vi "wrl_import_Ex.vi"() -> ()   [LabVIEW 2020]
uses:
  <vilib>/picture/3D Picture Control/Object/Create Object (name).vi
  Interface.vi
  <vilib>/picture/3D Picture Control/NI_3D Picture Control.lvlib
panel:
  out "3D 그림":refnum<vi>(3d-picture)
  in  "bkt angle":dbl
  in  "arm angle":dbl=0.07999999821186066
  in  "boom angle":dbl
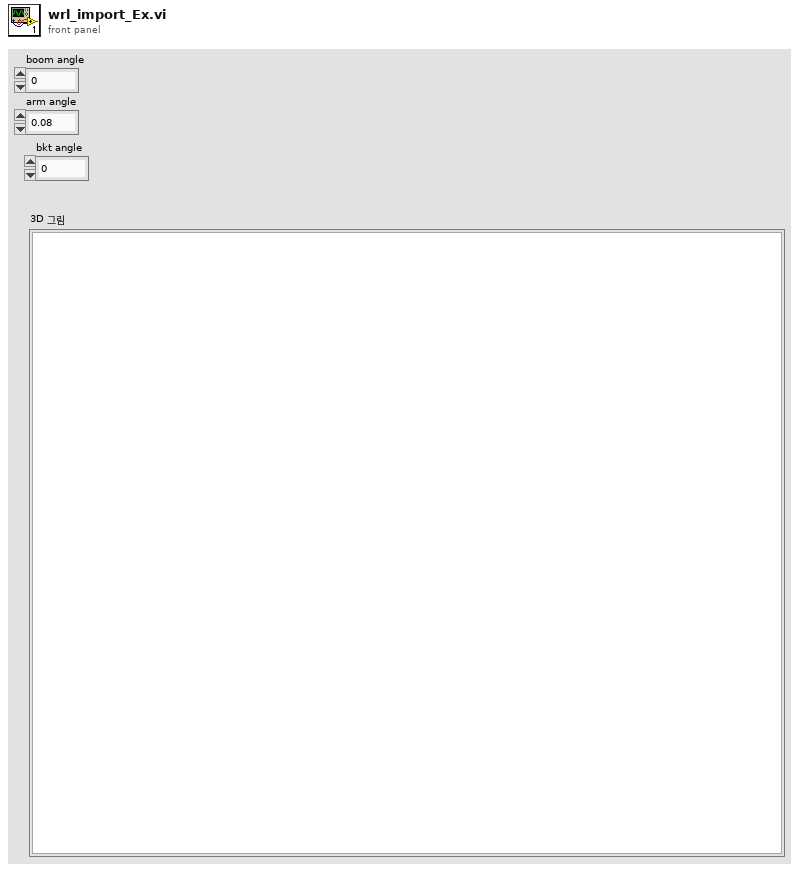
[diagram p1: front panel]
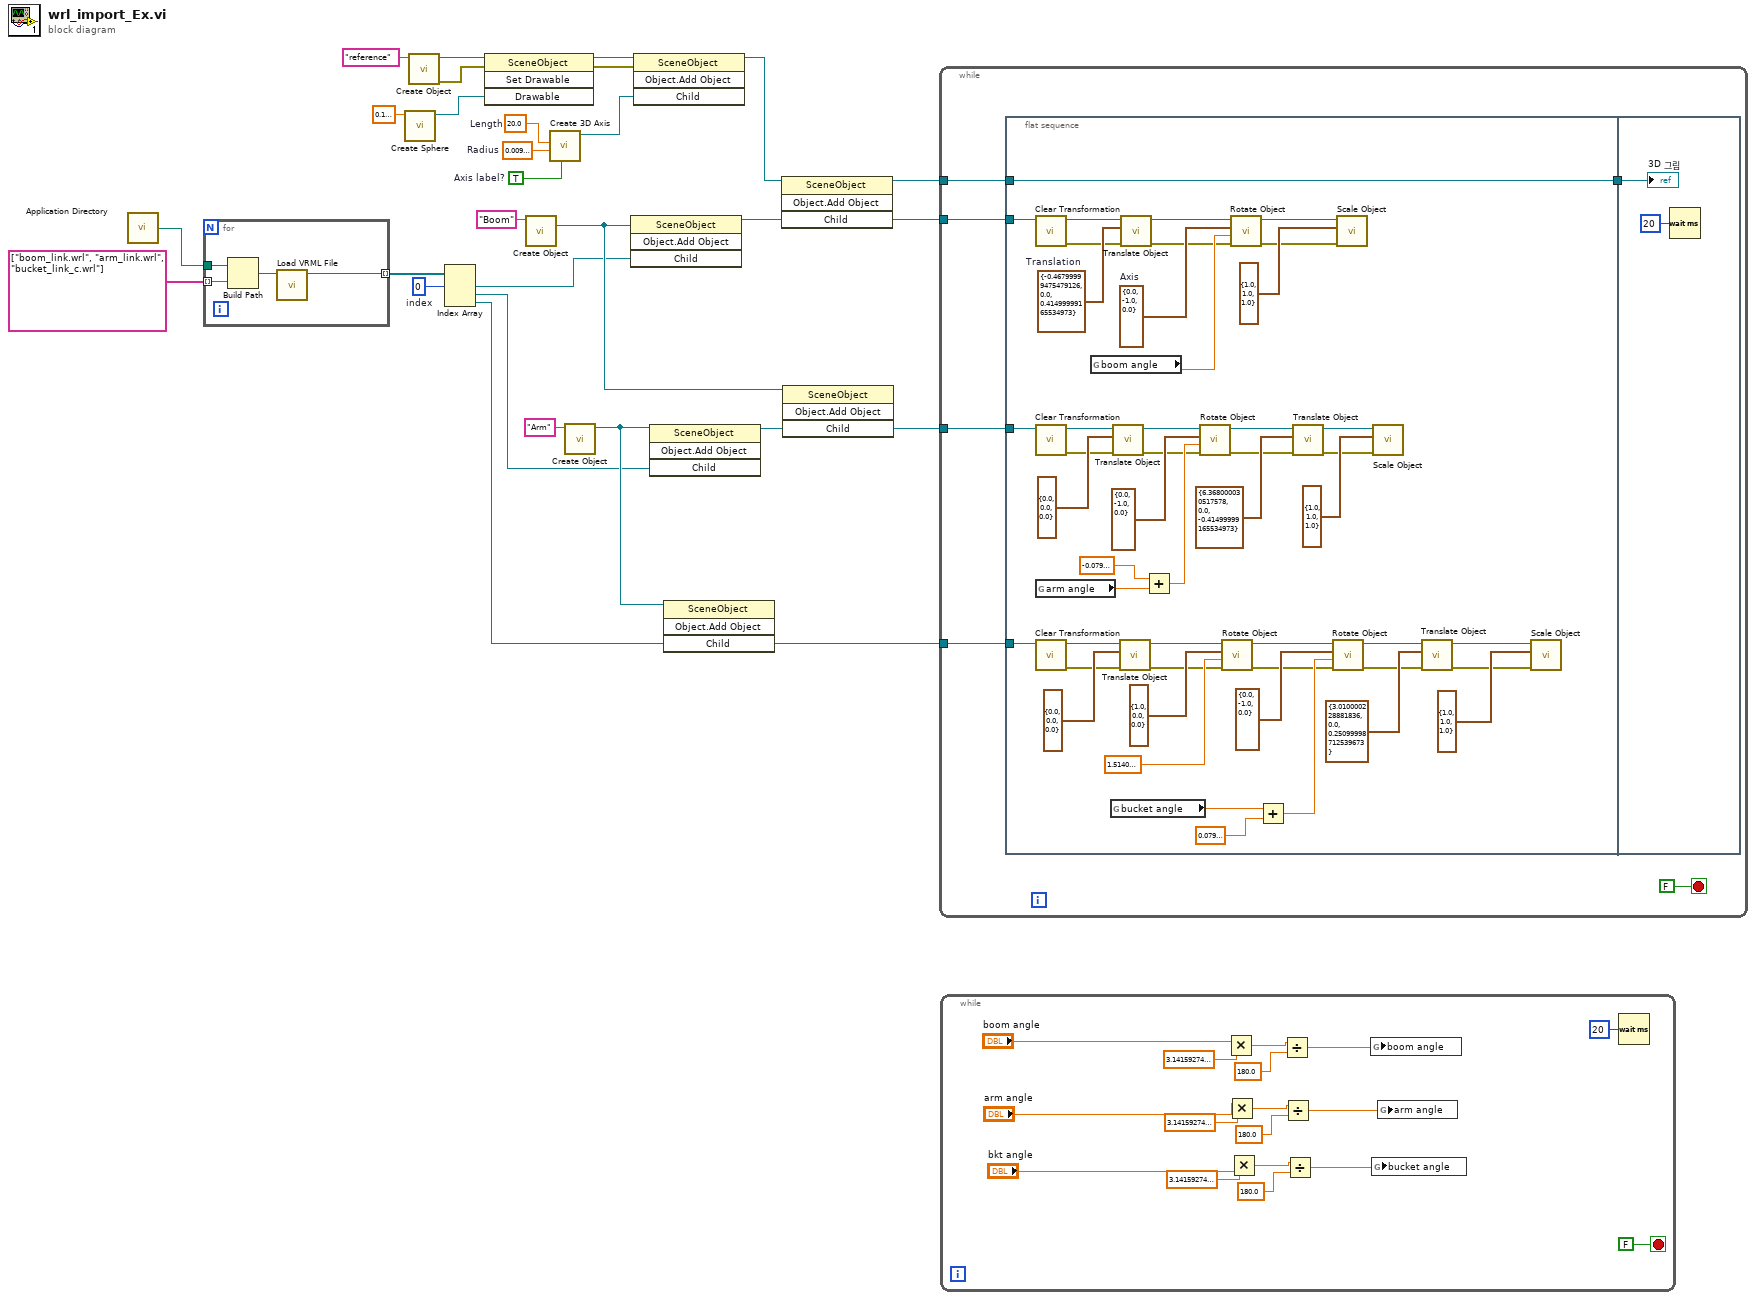
[diagram p0: block diagram]
diagram:
  w7 = 0  # index
  w15 = TRUE  # Axis label?
  w16 = sgl 0.01  # Radius
  w17 = sgl 20.0  # Length
  n1 = call <vilib>:"Application Directory.vi"() -> ("Application Directory"=w8:path)
  n2 = for {
    tunnel: string[] ["boom_link.wrl", "arm_link.wrl", "bucket_link_c.wrl"] -> [w33] mode=indexing
    tunnel: w8 -> [w32]
    tunnel: [w30] -> w5 mode=indexing
    n3 = Build Path(base path=w32, name or relative path=w33) -> (appended path=w31:path)
    n4 = call <vilib>:"Load VRML File.vi"("Path"=w31) -> ("Scene:Read Scene File"=w30:refnum<vi>)  [unwired: 9 in, 1 out]
  }
  n5 = call <vilib>:"Create Sphere.vi"("Radius"=sgl 0.1) -> ("New Sphere Refnum"=w26:refnum<vi>)  [unwired: 9 in, 1 out]
  n6 = call-poly <vilib>:"Create Object.vi"("Name"="reference") -> ("error out"=w2:errorcluster, "Scene:New Object"=w27:refnum<vi>)  [unwired: 9 in]
  n7 = Index Array "Index Array"(array=w5, index #1=w7) -> (element #1=w6:refnum<vi>, element #2=w4:refnum<vi>, element #3=w3:refnum<vi>)  [unwired: 2 in]
  n8 = invoke class="SceneObject" method="Set Drawable"(reference=w27, error in=w2, "Drawable"=w26) -> (reference out=w19:refnum<vi>, error out=w1:errorcluster)  [unwired: 1 in, 2 out]
  n9 = call-poly <vilib>:"Create Object.vi"("Name"="Boom") -> ("Scene:New Object"=w22:refnum<vi>)  [unwired: 9 in, 1 out]
  n10 = call <vilib>:"Create 3D Axis.vi"("Axis label?"=w15, "Radius"=w16, "Length"=w17) -> ("New Object Refnum"=w18:refnum<vi>)  [unwired: 7 in, 1 out]
  n11 = call-poly <vilib>:"Create Object.vi"("Name"="Arm") -> ("Scene:New Object"=w12:refnum<vi>)  [unwired: 9 in, 1 out]
  n12 = invoke class="SceneObject" method="Object.Add Object"(reference=w22, "Child"=w6) -> (reference out=w24:refnum<vi>)  [unwired: 2 in, 3 out]
  n13 = invoke class="SceneObject" method="Object.Add Object"(reference=w19, error in=w1, "Child"=w18) -> (reference out=w20:refnum<vi>)  [unwired: 1 in, 3 out]
  n14 = invoke class="SceneObject" method="Object.Add Object"(reference=w12, "Child"=w4) -> (reference out=w13:refnum<vi>)  [unwired: 2 in, 3 out]
  n15 = invoke class="SceneObject" method="Object.Add Object"(reference=w12, "Child"=w3) -> ("Child"=w10:refnum<vi>)  [unwired: 2 in, 3 out]
  n16 = invoke class="SceneObject" method="Object.Add Object"(reference=w20, "Child"=w24) -> (reference out=w25:refnum<vi>, "Child"=w21:refnum<vi>)  [unwired: 2 in, 2 out]
  n17 = invoke class="SceneObject" method="Object.Add Object"(reference=w22, "Child"=w13) -> ("Child"=w11:refnum<vi>)  [unwired: 2 in, 3 out]
  n18 = while {
    tunnel: w25 -> [w39]
    tunnel: w21 -> [w36]
    tunnel: w11 -> [w35]
    tunnel: w10 -> [w34]
    stop <- FALSE stop-if-true
    n19 = flat-sequence {
      tunnel: w39 -> [w87]
      tunnel: [w87] -> w37
      tunnel: w36 -> [w85]
      tunnel: w35 -> [w71]
      tunnel: w34 -> [w64]
      tunnel: w37 -> [w88]
      frame #0 {
        w86 = cluster{"X":sgl, "Y":sgl, "Z":sgl} {"X"=-0.468, "Y"=0.0, "Z"=0.415}  # Translation
        w81 = cluster{"X":sgl, "Y":sgl, "Z":sgl} {"X"=0.0, "Y"=-1.0, "Z"=0.0}  # Axis
        n20 = call <vilib>:"Clear Transformation.vi"("Object Refnum In"=w85) -> ("error out"=w51:errorcluster, "Object Refnum Out"=w84:refnum<vi>)  [unwired: 9 in]
        n21 = call <vilib>:"Clear Transformation.vi"("Object Refnum In"=w71) -> ("error out"=w43:errorcluster, "Object Refnum Out"=w79:refnum<vi>)  [unwired: 9 in]
        n22 = global read "Interface.vi" "arm angle"() -> (w58:dbl)
        n23 = call <vilib>:"Clear Transformation.vi"("Object Refnum In"=w64) -> ("error out"=w49:errorcluster, "Object Refnum Out"=w70:refnum<vi>)  [unwired: 9 in]
        n24 = global read "Interface.vi" "boom angle"() -> (w59:dbl)
        n25 = global read "Interface.vi" "bucket angle"() -> (w57:dbl)
        n26 = call <vilib>:"Translate Object.vi"("error in (no error)"=w43, "Translation"=cluster{"X":sgl, "Y":sgl, "Z":sgl} {"X"=0.0, "Y"=0.0, "Z"=0.0}, "Scene.Object In"=w79) -> ("error out"=w42:errorcluster, "Scene.Object Out"=w77:refnum<vi>)  [unwired: 7 in]
        n27 = call <vilib>:"Translate Object.vi"("error in (no error)"=w49, "Translation"=cluster{"X":sgl, "Y":sgl, "Z":sgl} {"X"=0.0, "Y"=0.0, "Z"=0.0}, "Scene.Object In"=w70) -> ("error out"=w48:errorcluster, "Scene.Object Out"=w55:refnum<vi>)  [unwired: 7 in]
        n28 = call <vilib>:"Translate Object.vi"("error in (no error)"=w51, "Translation"=w86, "Scene.Object In"=w84) -> ("error out"=w50:errorcluster, "Scene.Object Out"=w82:refnum<vi>)  [unwired: 7 in]
        n29 = Add(x=-0.07999999821186066 ("y"), y=w58) -> (x+y=w62:dbl)
        n30 = call <vilib>:"Rotate Object.vi"("error in (no error)"=w42, "Angle"=w62, "Axis"=cluster{"X":sgl, "Y":sgl, "Z":sgl} {"X"=0.0, "Y"=-1.0, "Z"=0.0}, "Scene.Object In"=w77) -> ("error out"=w41:errorcluster, "Scene.Object Out"=w73:refnum<vi>)  [unwired: 6 in]
        n31 = call <vilib>:"Rotate Object.vi"("error in (no error)"=w48, "Angle"=sgl 1.514, "Axis"=cluster{"X":sgl, "Y":sgl, "Z":sgl} {"X"=1.0, "Y"=0.0, "Z"=0.0}, "Scene.Object In"=w55) -> ("error out"=w47:errorcluster, "Scene.Object Out"=w53:refnum<vi>)  [unwired: 6 in]
        n32 = call <vilib>:"Rotate Object.vi"("error in (no error)"=w50, "Angle"=w59, "Axis"=w81, "Scene.Object In"=w82) -> ("error out"=w44:errorcluster, "Scene.Object Out"=w80:refnum<vi>)  [unwired: 6 in]
        n33 = Add(x=w57, y=0.07999999821186066) -> (x+y=w60:dbl)
        n34 = call <vilib>:"Translate Object.vi"("error in (no error)"=w41, "Translation"=cluster{"X":sgl, "Y":sgl, "Z":sgl} {"X"=6.368, "Y"=0.0, "Z"=-0.415}, "Scene.Object In"=w73) -> ("error out"=w40:errorcluster, "Scene.Object Out"=w72:refnum<vi>)  [unwired: 7 in]
        n35 = call <vilib>:"Rotate Object.vi"("error in (no error)"=w47, "Angle"=w60, "Axis"=cluster{"X":sgl, "Y":sgl, "Z":sgl} {"X"=0.0, "Y"=-1.0, "Z"=0.0}, "Scene.Object In"=w53) -> ("error out"=w46:errorcluster, "Scene.Object Out"=w66:refnum<vi>)  [unwired: 6 in]
        n36 = call <vilib>:"Scale Object.vi"("error in (no error)"=w44, "Scale"=cluster{"X":sgl, "Y":sgl, "Z":sgl} {"X"=1.0, "Y"=1.0, "Z"=1.0}, "Scene.Object In"=w80) -> ()  [unwired: 7 in, 2 out]
        n37 = call <vilib>:"Scale Object.vi"("error in (no error)"=w40, "Scale"=cluster{"X":sgl, "Y":sgl, "Z":sgl} {"X"=1.0, "Y"=1.0, "Z"=1.0}, "Scene.Object In"=w72) -> ()  [unwired: 7 in, 2 out]
        n38 = call <vilib>:"Translate Object.vi"("error in (no error)"=w46, "Translation"=cluster{"X":sgl, "Y":sgl, "Z":sgl} {"X"=3.0100002, "Y"=0.0, "Z"=0.251}, "Scene.Object In"=w66) -> ("error out"=w45:errorcluster, "Scene.Object Out"=w65:refnum<vi>)  [unwired: 7 in]
        n39 = call <vilib>:"Scale Object.vi"("error in (no error)"=w45, "Scale"=cluster{"X":sgl, "Y":sgl, "Z":sgl} {"X"=1.0, "Y"=1.0, "Z"=1.0}, "Scene.Object In"=w65) -> ()  [unwired: 7 in, 2 out]
      }
      frame #1 {
        n40 = Wait (ms)(milliseconds to wait=u32 20 ("대기 시간 (ms)")) -> ()  [unwired: 1 out]
        "3D 그림" <- w88
      }
    }
  }
  n41 = while {
    stop <- FALSE stop-if-true
    n42 = Multiply(x="boom angle", y=3.1415927410125732) -> (x*y=w102:dbl)
    n43 = Multiply(x="arm angle", y=3.1415927410125732) -> (x*y=w98:dbl)
    n44 = Multiply(x="bkt angle", y=3.1415927410125732) -> (x*y=w94:dbl)
    n45 = Divide(x=w102, y=180.0) -> (x/y=w100:dbl)
    n46 = Divide(x=w98, y=180.0) -> (x/y=w96:dbl)
    n47 = Divide(x=w94, y=180.0) -> (x/y=w92:dbl)
    n48 = global write "Interface.vi" "boom angle"(w100) -> ()
    n49 = global write "Interface.vi" "bucket angle"(w92) -> ()
    n50 = global write "Interface.vi" "arm angle"(w96) -> ()
    n51 = Wait (ms)(milliseconds to wait=u32 20 ("대기 시간 (ms)")) -> ()  [unwired: 1 out]
  }
